vi "temperature monitoring.vi"() -> ()   [LabVIEW 2026]
panel:
  in  "Fill Color":u32(colorbox)
  out "Value is higher":bool
  in  "Enter the higher Temp":i32
  out "Thermometer":dbl(slide) scale=0.0..100.0
  out "String":string
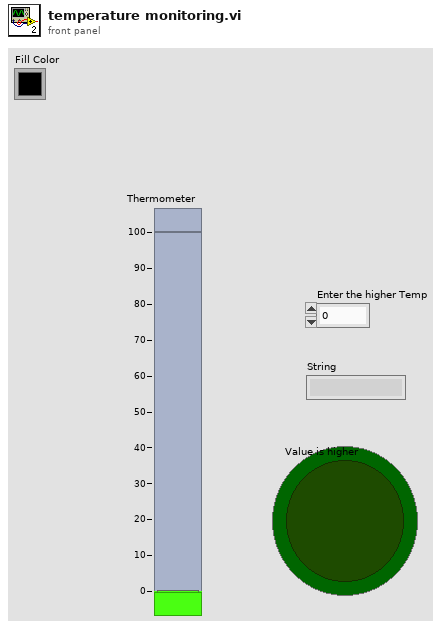
[diagram p1: front panel]
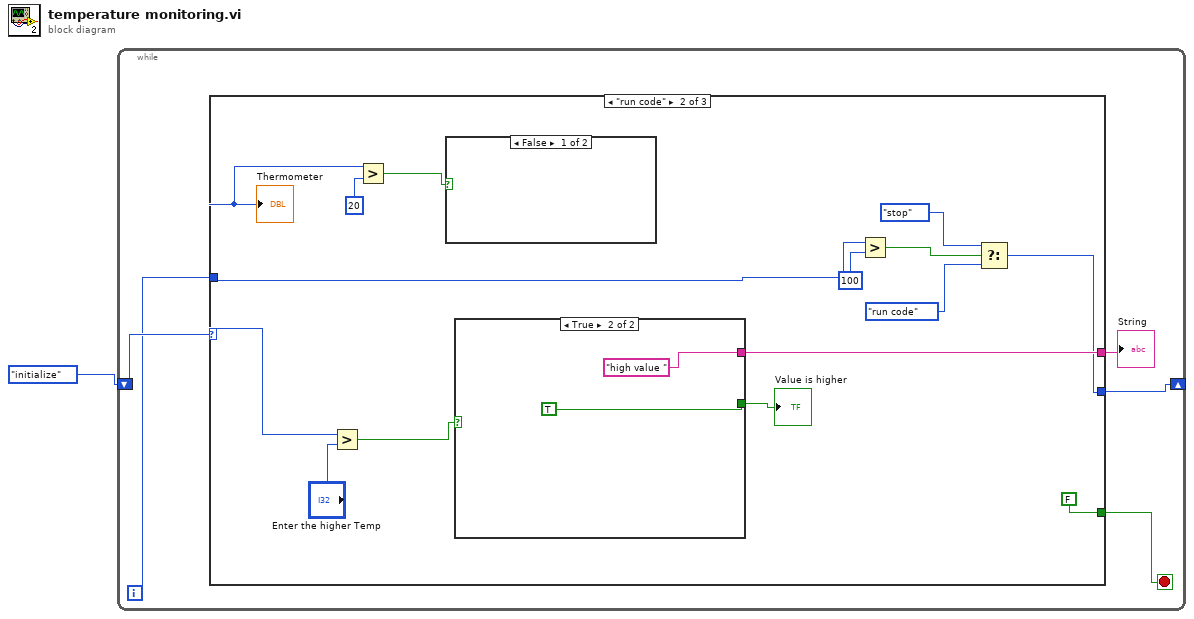
[diagram p0: block diagram]
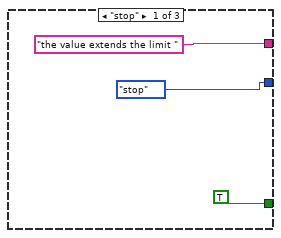
[diagram p2: hidden frame]
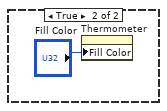
[diagram p3: hidden frame]
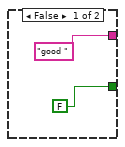
[diagram p4: hidden frame]
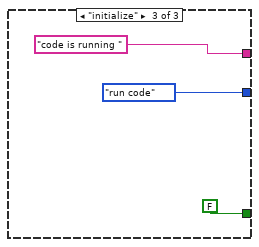
[diagram p5: hidden frame]
diagram:
  n1 = while {
    shift-right: [w2] -> _
    shift-left: enum16{"stop", "run code", "initialize"}."initialize" -> [w6]
    i -> [w3]
    stop <- w5 stop-if-true
    n2 = case shown="\"run code\"" w6 {
      tunnel: [TRUE ("stop") FALSE ("stop") FALSE ("stop")] -> w5
      tunnel: ["the value extends the limit " w18 "code is running "] -> w4
      tunnel: w3 -> [_ w12 _]
      tunnel: [enum16{"stop", "run code", "initialize"}."stop" w13 enum16{"stop", "run code", "initialize"}."run code"] -> w2
      frame "stop" {
      }
      frame "run code" {
        n3 = Greater?(x=w12, y="Enter the higher Temp") -> (0:w21:bool)
        n4 = Greater?(x=w12, y=20) -> (0:w10:bool)
        n5 = case shown="False" w10 {
          frame False {
          }
          frame True {
            n6 = property on="Thermometer" class="Slide (strict)"("Fill Color"="Fill Color") -> ()  [unwired: 2 in, 2 out]
          }
        }
        n7 = case shown="True" w21 {
          tunnel: [FALSE TRUE] -> w20
          tunnel: ["good " "high value "] -> w18
          frame False {
          }
          frame True {
          }
        }
        "Value is higher" <- w20
        n8 = Greater?(x=w12, y=100) -> (0:w16:bool)
        n9 = Select(t=enum16{"stop", "run code", "initialize"}."stop", s=w16, f=enum16{"stop", "run code", "initialize"}."run code") -> (s? t:f=w13:enum16{"stop", "run code", "initialize"})
        "Thermometer" <- w12
      }
      frame "initialize" {
      }
    }
    "String" <- w4
  }
